vi "PID_model_02.vi"() -> ()   [LabVIEW 2022 SP3]
uses:
  <vilib>/Platform/TimedLoop/XDataNode/timing_clust.ctl
  <vilib>/Platform/TimedLoop/XDataNode/nitl_modes.ctl
  <vilib>/Platform/TimedLoop/XDataNode/wakeup.ctl
  <vilib>/Utility/file.llb/Read Delimited Spreadsheet (DBL).vi
  <vilib>/Platform/TimedLoop/scheduler/LVUserAPI/_suppVIs/Create_1kHz_TSource.vi
  <vilib>/platform/TimedLoop/XDataNode/XDataNode.xnode
  <vilib>/Platform/TimedLoop/XDataNode/XDNodeRunTimeDep.lvlib
  <vilib>/addons/control/pid/NI_PID_pid.lvlib
  <vilib>/gmath/NI_Gmath.lvlib
  <vilib>/addons/control/pid/pid.llb/PID (DBL).vi
panel:
  in  "method":i32(ring)=1 items=["nearest", "linear", "spline", "cubic Hermite", "Lagrange"]
  in  "cluster 2":T1={"Initial X Axis Value"=0, "X Axis Increment"=6.10352, []}
  in  "Setpoint 2":dbl
  in  "Proportional Gain 2":dbl
  in  "method 2":i32(ring)=1 items=["nearest", "linear", "spline", "cubic Hermite", "Lagrange"]
  in  "stop":bool
  out "Plant Output":dbl[](graph)
  in  "cluster":T1={"Initial X Axis Value"=0, "X Axis Increment"=6.10352, []}
  out "Excitation & Response FRFs":T2(graph)
  out "Phase 2":cluster{"Array":dbl[], "Array":dbl[]}(graph) caption="Amplitude [Hz]"
  in  "Skip First N Lines 2":i32=48
  out "Magnitude 2":cluster{"Array":dbl[], "Array":dbl[]}(graph) caption="Amplitude [Hz]"
  out "number of rows 2":i32
  in  "name or relative path 2":path=path "C:/Users/LAV-UFSC/OneDrive - UFSC/Documents/LAV - TCC/Dados-Experimentos/25-04/frf_8.txt"
  out "Phase":cluster{"Array":dbl[], "Array":dbl[]}(graph) caption="Amplitude [Hz]"
  in  "Skip First N Lines":i32=48
  out "Magnitude":cluster{"Array":dbl[], "Array":dbl[]}(graph) caption="Amplitude [Hz]"
  out "number of rows":i32
  in  "name or relative path":path=path "C:/Users/LAV-UFSC/OneDrive - UFSC/Documents/LAV - TCC/Dados-Experimentos/25-04/frf_3.txt"
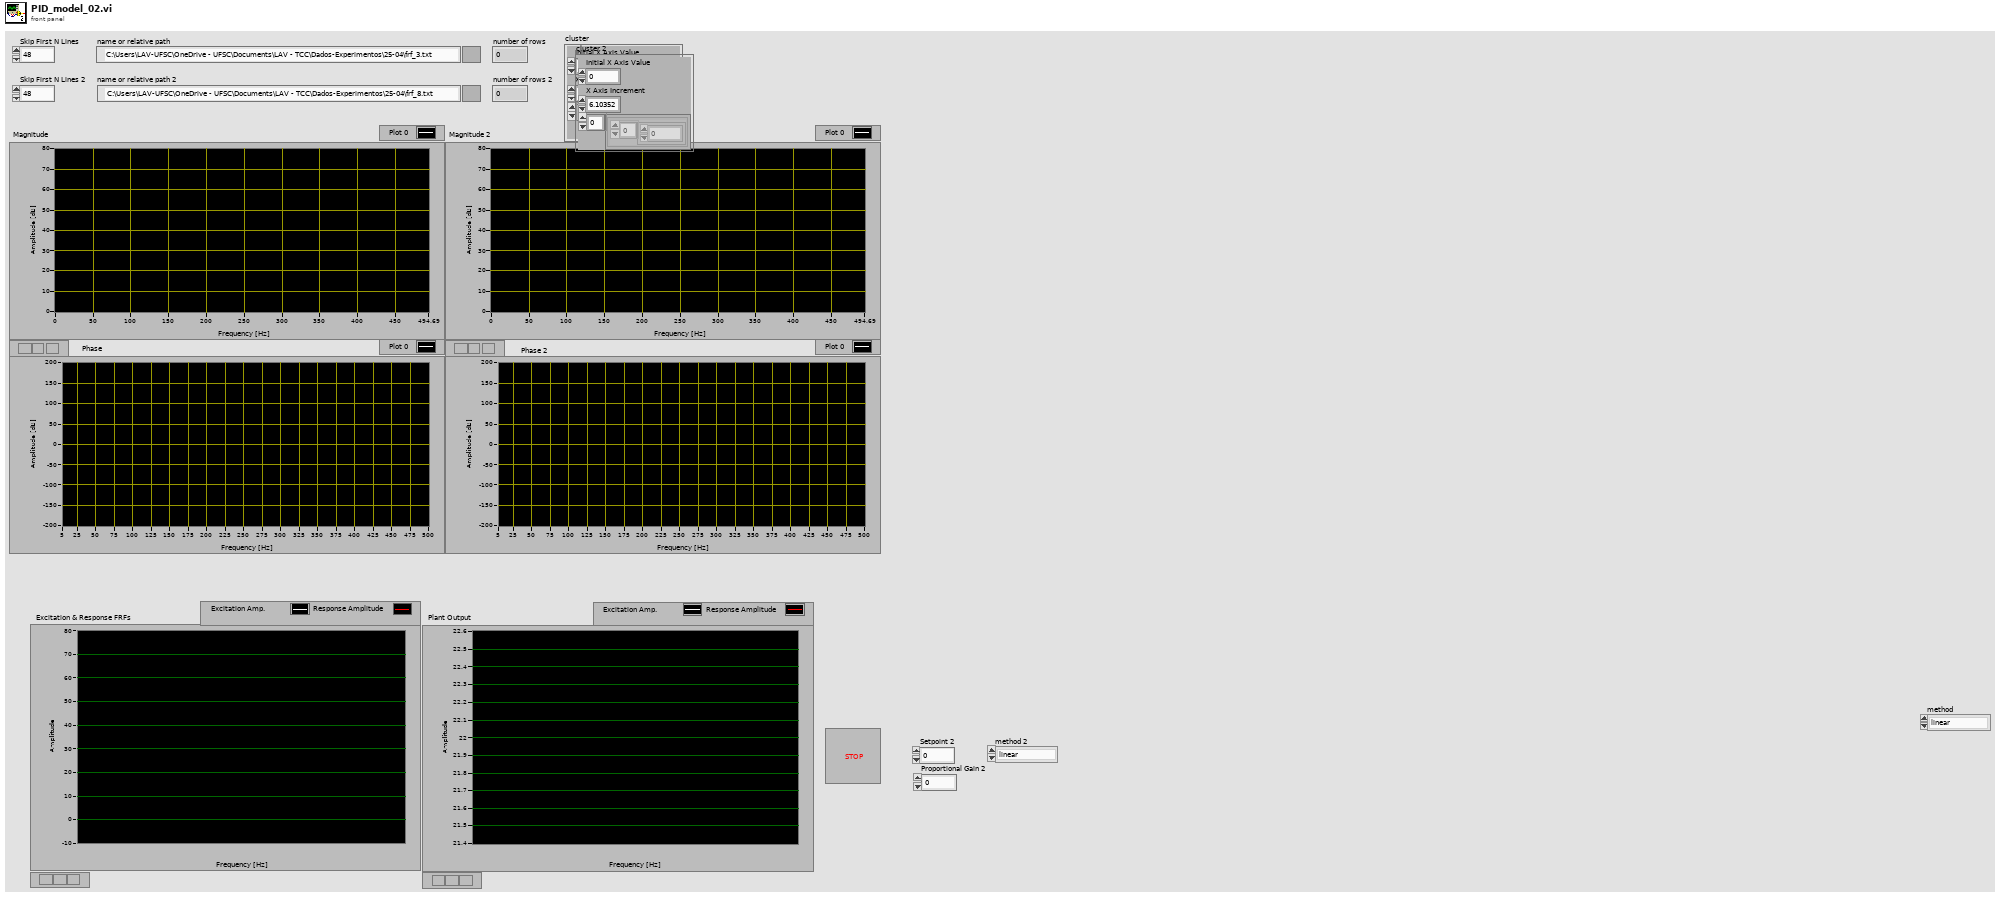
[diagram p1: front panel]
types:
  T1 = cluster{"Initial X Axis Value":i32, "X Axis Increment":dbl, cluster{dbl[]}[]}
  T2 = cluster{i32, "X Axis Increment":dbl, cluster{dbl[]}[]}
  T3 = typedef "XDNodeRunTimeDep.lvlib/timing_clust.ctl" = cluster{"Expected End [f-1]":u64, "Actual End [f-1]":u64, "Finished Late? [f-1]":bool, "Expected End [i-1]":u64, "Actual End [i-1]":u64, "Finished Late? [i-1]":bool, "Expected Start [i]":u64, "Actual Start [i]":u64, "Expected Start [f]":u64, "Actual Start [f]":u64, "Source Name":string, "Structure Name":string, "Period":i64, "Deadline":i64, "Offset":i64, "Start":i64, "Priority":i32, "Timeout":i32, "Mode":T4, "Wakeup Reason":T5, "Error":errorcluster, "Source Type":string, "Secondary Source Type":string, "Global End Time":u64, "Global Start Time":u64, "Frame Duration":u64, "Iteration Duration":u64, "Assigned CPU":i32, "I/O Scan Engine Mode":u32}
  T4 = typedef "XDNodeRunTimeDep.lvlib/nitl_modes.ctl" = enum32{"No Change", "Process missed periods, maintain original phase", "Discard missed periods, maintain original phase", "Process missed periods, ignore original phase", "Discard missed periods, ignore original phase"}
  T5 = typedef "XDNodeRunTimeDep.lvlib/wakeup.ctl" = enum32{"Normal", "Aborted", "Asynchronous wakeup", "Timing source error", "Timed loop error", "Timeout"}
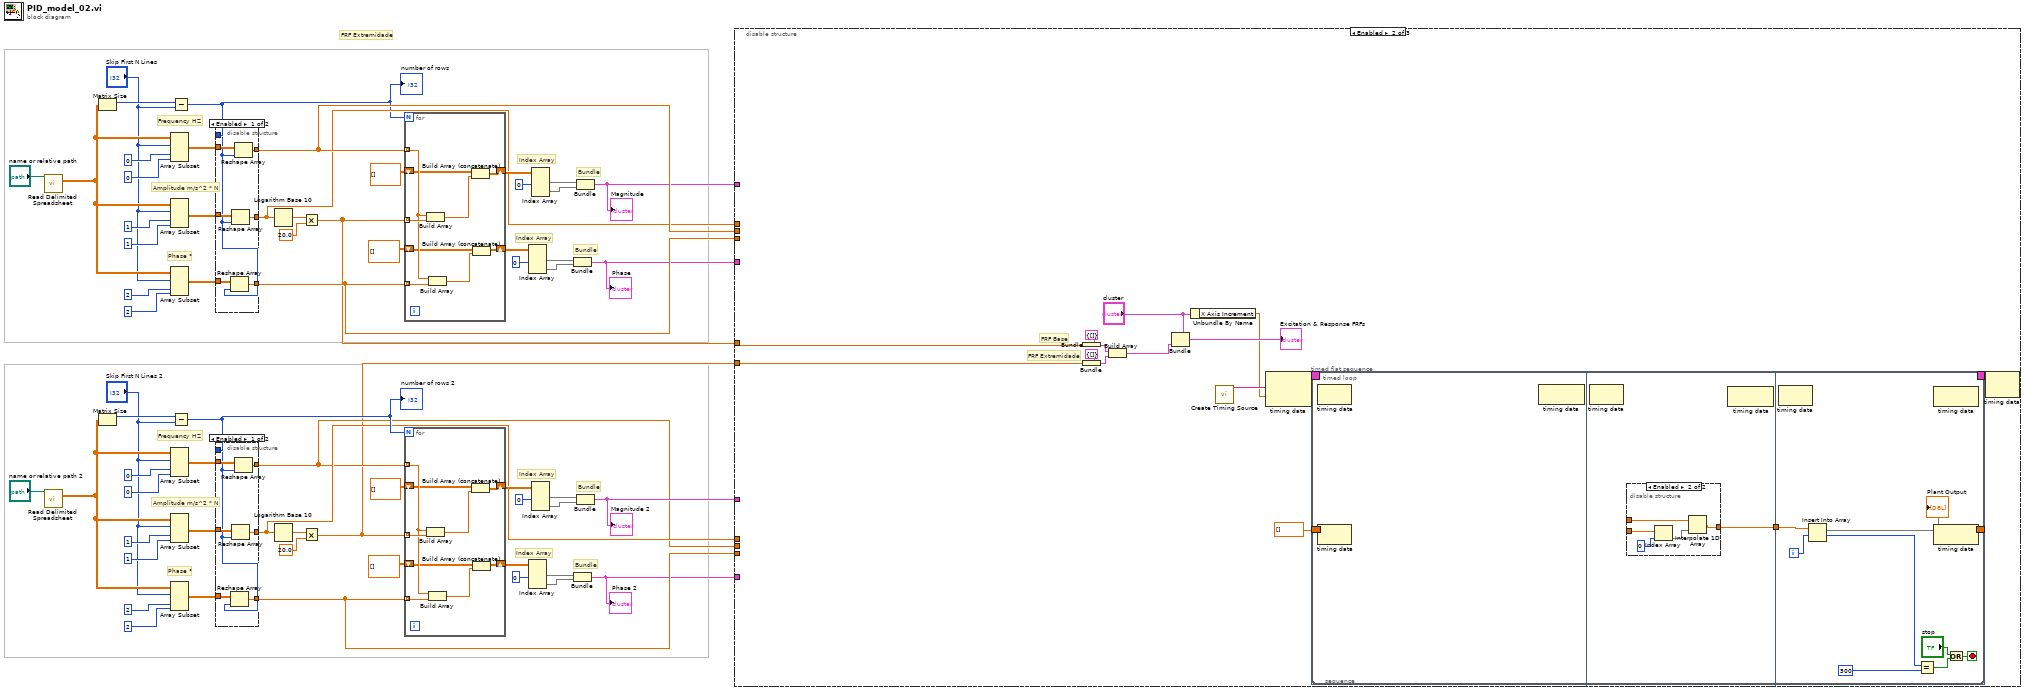
[diagram p0: block diagram]
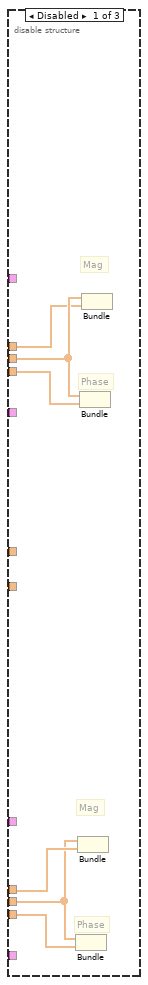
[diagram p3: hidden frame]
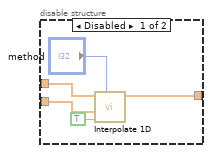
[diagram p4: hidden frame]
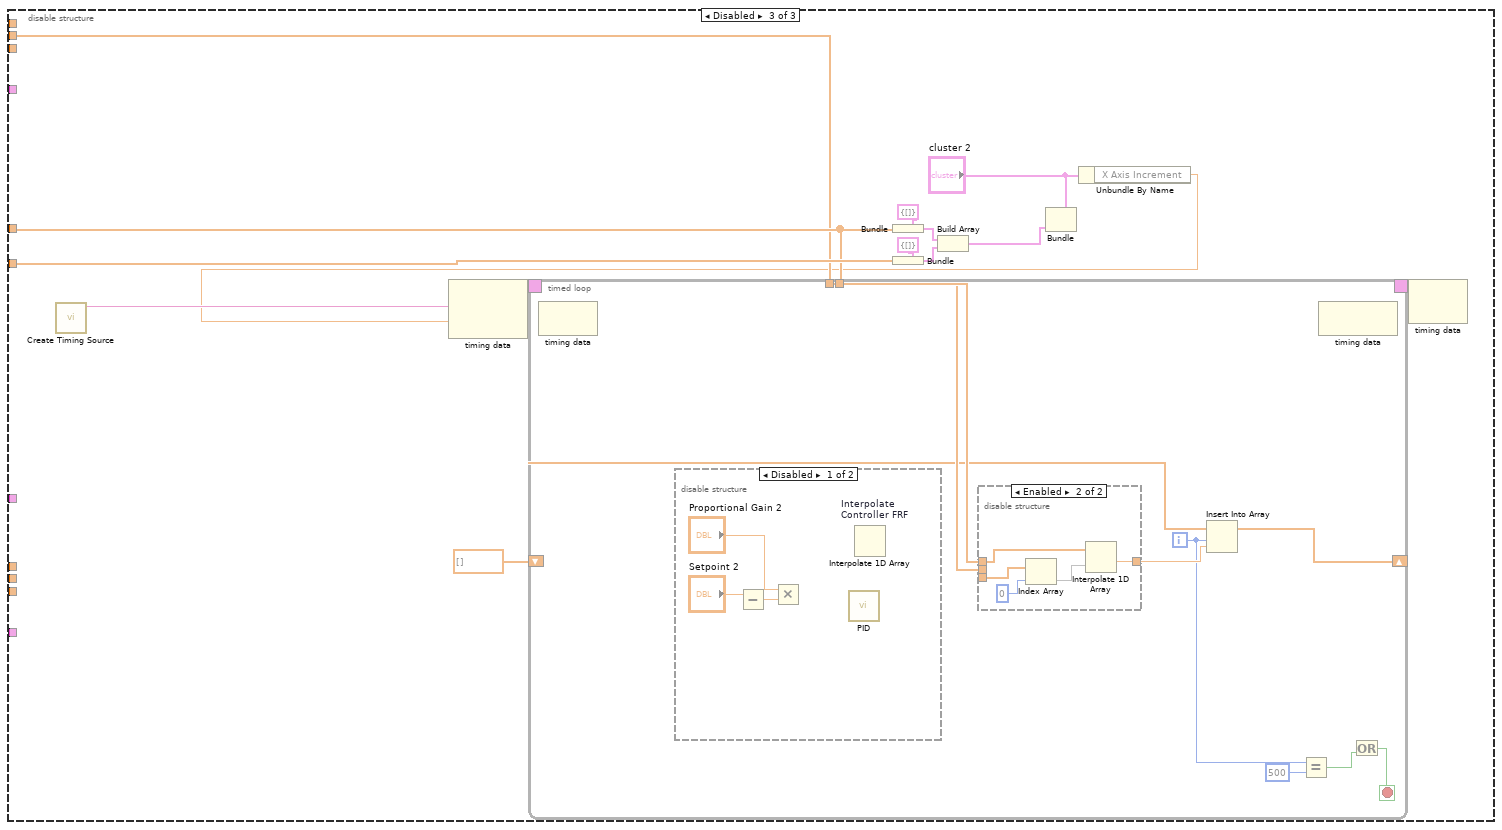
[diagram p5: hidden frame]
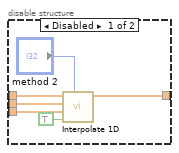
[diagram p6: hidden frame]
diagram:
  # "Index Array"
  # "Bundle"
  # "Index Array"
  # "Bundle"
  # "Phase °"
  # "Amplitude m/s^2 * N"
  # "Frequency HZ"
  # "FRF Extremidade"
  # "Index Array"
  # "Bundle"
  # "Index Array"
  # "Bundle"
  # "Phase °"
  # "Amplitude m/s^2 * N"
  # "Frequency HZ"
  n1 = call-poly <vilib>:"Read Delimited Spreadsheet.vi"("file path (dialog if empty)"="name or relative path") -> ("all rows"=w55:dbl[][])  [unwired: 9 in, 5 out]
  n2 = call-poly <vilib>:"Read Delimited Spreadsheet.vi"("file path (dialog if empty)"="name or relative path 2") -> ("all rows"=w24:dbl[][])  [unwired: 9 in, 5 out]
  n3 = Matrix Size(0:w55) -> (1:w38:i32)  [unwired: 1 out]
  n4 = Matrix Size(0:w24) -> (1:w10:i32)  [unwired: 1 out]
  n5 = Array Subset(array=w55, index (row)="Skip First N Lines", index (col)=0 ("column 1"), length (col)=0 ("column N")) -> (w57:dbl[][])  [unwired: 1 in]
  n6 = Array Subset(array=w55, index (row)="Skip First N Lines", index (col)=1 ("column 1"), length (col)=1 ("column N")) -> (w56:dbl[][])  [unwired: 1 in]
  n7 = Array Subset(array=w55, index (row)="Skip First N Lines", index (col)=2 ("column 1"), length (col)=2 ("column N")) -> (w40:dbl[][])  [unwired: 1 in]
  n8 = Array Subset(array=w24, index (row)="Skip First N Lines 2", index (col)=0 ("column 1"), length (col)=0 ("column N")) -> (w26:dbl[][])  [unwired: 1 in]
  n9 = Array Subset(array=w24, index (row)="Skip First N Lines 2", index (col)=1 ("column 1"), length (col)=1 ("column N")) -> (w25:dbl[][])  [unwired: 1 in]
  n10 = Array Subset(array=w24, index (row)="Skip First N Lines 2", index (col)=2 ("column 1"), length (col)=2 ("column N")) -> (w11:dbl[][])  [unwired: 1 in]
  n11 = Subtract(x=w38, y="Skip First N Lines") -> (x-y=w36:i32)
  "number of rows" <- w36
  n12 = Subtract(x=w10, y="Skip First N Lines 2") -> (x-y=w8:i32)
  "number of rows 2" <- w8
  n13 = disable-structure shown="Enabled" {
    disable-tunnel: w57 -> [w71 w73]
    disable-tunnel: w56 -> [w70 w72]
    disable-tunnel: [w69 w73] -> w42
    disable-tunnel: [w68 w72] -> w41
    disable-tunnel: w36 -> [w66 _]
    disable-tunnel: w40 -> [w67 _]
    disable-tunnel: [w65 _] -> w39
    frame Enabled {
      n14 = Reshape Array(w67, w66) -> (w65:dbl[])
      n15 = Reshape Array(w70, w66) -> (w68:dbl[])
      n16 = Reshape Array(w71, w66) -> (w69:dbl[])
    }
    frame Disabled {
    }
  }
  n17 = disable-structure shown="Enabled" {
    disable-tunnel: w26 -> [w80 w82]
    disable-tunnel: w25 -> [w79 w81]
    disable-tunnel: [w78 w82] -> w5
    disable-tunnel: [w77 w81] -> w6
    disable-tunnel: w8 -> [w75 _]
    disable-tunnel: w11 -> [w76 _]
    disable-tunnel: [w74 _] -> w4
    frame Enabled {
      n18 = Reshape Array(w76, w75) -> (w74:dbl[])
      n19 = Reshape Array(w79, w75) -> (w77:dbl[])
      n20 = Reshape Array(w80, w75) -> (w78:dbl[])
    }
    frame Disabled {
    }
  }
  n21 = Logarithm Base 10(1:w41) -> (0:w48:dbl[])
  n22 = Logarithm Base 10(1:w6) -> (0:w17:dbl[])
  n23 = Multiply(x=w48, y=20.0) -> (x*y=w1:dbl[])
  n24 = Multiply(x=w17, y=20.0) -> (x*y=w2:dbl[])
  n25 = for {
    N: w36 -> [_]
    tunnel: w42 -> [w89] mode=indexing
    tunnel: w1 -> [w90] mode=indexing
    tunnel: w39 -> [w91] mode=indexing
    shift-right: [w86] -> w50
    shift-left: dbl[][] [] -> [w88]
    shift-right: [w85] -> w43
    shift-left: dbl[][] [] -> [w84]
    n26 = Build Array(w89, w90) -> (w87:dbl[])
    n27 = Build Array(w89, w91) -> (w83:dbl[])
    n28 = Build Array (concatenate)(w88, w87) -> (w86:dbl[][])
    n29 = Build Array (concatenate)(w84, w83) -> (w85:dbl[][])
  }
  n30 = for {
    N: w8 -> [_]
    tunnel: w5 -> [w98] mode=indexing
    tunnel: w2 -> [w99] mode=indexing
    tunnel: w4 -> [w100] mode=indexing
    shift-right: [w95] -> w19
    shift-left: dbl[][] [] -> [w97]
    shift-right: [w94] -> w12
    shift-left: dbl[][] [] -> [w93]
    n31 = Build Array(w98, w99) -> (w96:dbl[])
    n32 = Build Array(w98, w100) -> (w92:dbl[])
    n33 = Build Array (concatenate)(w97, w96) -> (w95:dbl[][])
    n34 = Build Array (concatenate)(w93, w92) -> (w94:dbl[][])
  }
  n35 = Index Array(array=w43, index (col) #1=0 ("disabled index (col)")) -> (element #1=w44:dbl[], element #2=w45:dbl[])  [unwired: 3 in]
  n36 = Index Array(array=w12, index (col) #1=0 ("disabled index (col)")) -> (element #1=w13:dbl[], element #2=w14:dbl[])  [unwired: 3 in]
  n37 = Index Array(array=w50, index (col) #1=0 ("disabled index (col)")) -> (element #1=w51:dbl[], element #2=w52:dbl[])  [unwired: 3 in]
  n38 = Index Array(array=w19, index (col) #1=0 ("disabled index (col)")) -> (element #1=w20:dbl[], element #2=w21:dbl[])  [unwired: 3 in]
  n39 = Bundle(w44, w45) -> (w34:cluster{dbl[], dbl[]})  [unwired: 1 in]
  "Phase" <- w34
  n40 = Bundle(w13, w14) -> (w3:cluster{dbl[], dbl[]})  [unwired: 1 in]
  "Phase 2" <- w3
  n41 = Bundle(w51, w52) -> (w35:cluster{dbl[], dbl[]})  [unwired: 1 in]
  "Magnitude" <- w35
  n42 = Bundle(w20, w21) -> (w7:cluster{dbl[], dbl[]})  [unwired: 1 in]
  "Magnitude 2" <- w7
  n43 = disable-structure shown="Enabled" {
    disable-tunnel: w42 -> [w106 _ w162]
    disable-tunnel: w41 -> [w105 _ _]
    disable-tunnel: w39 -> [w104 _ _]
    disable-tunnel: w35 -> [_ _ _]
    disable-tunnel: w34 -> [_ _ _]
    disable-tunnel: w7 -> [_ _ _]
    disable-tunnel: w6 -> [w103 _ _]
    disable-tunnel: w5 -> [w101 _ _]
    disable-tunnel: w4 -> [w102 _ _]
    disable-tunnel: w3 -> [_ _ _]
    disable-tunnel: w2 -> [_ w116 w168]
    disable-tunnel: w1 -> [_ w113 w165]
    frame Disabled {
      # "Phase"
      # "Mag"
      # "Phase"
      # "Mag"
      n44 = Bundle("all rows"=w101, "all rows"=w102) -> ()  [unwired: 2 out]
      n45 = Bundle("all rows"=w101, "all rows"=w103) -> ()  [unwired: 2 out]
      n46 = Bundle("all rows"=w106, "all rows"=w104) -> ()  [unwired: 2 out]
      n47 = Bundle("all rows"=w106, "all rows"=w105) -> ()  [unwired: 2 out]
    }
    frame Enabled {
      # "FRF Base"
      # "FRF Extremidade"
      n48 = Bundle(cluster=cluster{dbl[]} {[]} ("Excitation Amplitude [dB]"), w113) -> (w120:cluster{dbl[]})
      n49 = Bundle(cluster=cluster{dbl[]} {[]} ("Response Amplitude [dB]"), w116) -> (w119:cluster{dbl[]})
      n50 = Build Array(w120, w119) -> (w118:cluster{dbl[]}[])
      n51 = Bundle(cluster="cluster", w118) -> (→"Excitation & Response FRFs":T1)  [unwired: 2 in]
      n52 = Unbundle By Name("cluster") -> ("X Axis Increment"=w108:dbl)
      n53 = call-poly <vilib>:"Create Timing Source.vi"() -> ("name (out)"=w109:string)  [unwired: 10 in, 1 out]
      n54 = node-c288(w109, w108) -> (w112:T3)
      n55 = timed-loop {
        timing: w112 -> [_]
        timing-out: [_] -> w111
        shift-right: [w121] -> _
        shift-left: dbl[] [] ("yi") -> [w122]
        i -> [w147]
        stop <- w144 stop-if-true
        n56 = timed-sequence {
          timing: _ -> [_]
          timing-out: _ -> [_]
          tunnel: w122 -> [w125]
          tunnel: [w124] -> w121
          n57 = timed-flat-sequence {
            tunnel: w125 -> [_]
            tunnel: [w128] -> w123
            tunnel: [w143] -> w124
            tunnel: w123 -> [w142]
            frame #0 {
              n58 = node-c288() -> ()  [unwired: 1 in, 1 out]
              n59 = node-c288() -> ()  [unwired: 1 in, 1 out]
            }
            frame #1 {
              n60 = node-c288() -> ()  [unwired: 1 in, 1 out]
              n61 = disable-structure shown="Enabled" {
                disable-tunnel: _ -> [w134 w138]
                disable-tunnel: _ -> [w131 w137]
                disable-tunnel: [w130 w139] -> w128
                frame Disabled {
                  n62 = call <vilib>:"Interpolate 1D.vi"("method"="method", "X is monotonic"=TRUE, "xi"=w131, "Y"=w134) -> ("yi"=w130:dbl[], "X"=w133:dbl[])  [unwired: 4 in, 2 out]
                }
                frame Enabled {
                  n63 = Index Array(array=w137, index=0) -> (element=w135)
                  n64 = Interpolate 1D Array(1:w135, 2:w138) -> (0:w139:dbl)
                }
              }
              n65 = node-c288() -> ()  [unwired: 1 in, 1 out]
            }
            frame #2 {
              n66 = node-c288() -> ()  [unwired: 1 in, 1 out]
              n67 = Insert Into Array(array=w142, index=w147) -> (w143)  [unwired: 1 in]
              "Plant Output" <- w143
              n68 = Equal?(x=w147, y=500) -> (x = y?=w146:bool)
              n69 = node-c288() -> ()  [unwired: 1 in, 1 out]
              n70 = Or(x="stop", y=w146) -> (x .or. y?=w144:bool)
            }
          }
        }
        n71 = node-c288() -> ()  [unwired: 1 in, 1 out]
        n72 = node-c288() -> ()  [unwired: 1 in, 1 out]
      }
      n73 = node-c288(w111) -> ()  [unwired: 1 out]
    }
    frame Disabled {
      n74 = call-poly <vilib>:"Create Timing Source.vi"() -> ("name (out)"=w160:string)  [unwired: 10 in, 1 out]
      n75 = Bundle(cluster=cluster{dbl[]} {[]} ("Excitation Amplitude [dB]"), w165) -> (w172:cluster{dbl[]})
      n76 = Bundle(cluster=cluster{dbl[]} {[]} ("Response Amplitude [dB]"), w168) -> (w171:cluster{dbl[]})
      n77 = Build Array(w172, w171) -> (w170:cluster{dbl[]}[])
      n78 = Bundle(cluster="cluster 2", w170) -> (w169:T1)  [unwired: 2 in]
      n79 = Unbundle By Name("cluster 2") -> ("X Axis Increment"=w159:dbl)
      n80 = node-c288(w160, w159) -> (w164:T3)
      n81 = timed-loop {
        tunnel: w165 -> [w181]
        timing: w164 -> [_]
        timing-out: [_] -> w163
        tunnel: w162 -> [w180]
        shift-right: [w178] -> _
        shift-left: dbl[] [] ("yi") -> [w179]
        i -> [w174]
        stop <- w176 stop-if-true
        n82 = node-c288() -> ()  [unwired: 1 in, 1 out]
        n83 = disable-structure shown="Disabled" {
          frame Disabled {
            n84 = Subtract(x="Setpoint 2") -> (y=w193:dbl, x-y=w195:dbl)
            n85 = Multiply(x="Proportional Gain 2", y=w195) -> ()  [unwired: 1 out]
            n86 = call-poly <vilib>:"PID.vi"() -> ()  [unwired: 10 in, 2 out]
            n87 = Interpolate 1D Array "Interpolate\nController FRF"() -> ()  [unwired: 2 in, 1 out]
          }
          frame Enabled {
          }
        }
        n88 = disable-structure shown="Enabled" {
          disable-tunnel: w181 -> [w187 w191]
          disable-tunnel: w180 -> [w186 _]
          disable-tunnel: _ -> [w184 w190]
          disable-tunnel: [w183 w192] -> w177
          frame Disabled {
            n89 = call <vilib>:"Interpolate 1D.vi"("method"="method 2", "X is monotonic"=TRUE, "xi"=w184, "X"=w186, "Y"=w187) -> ("yi"=w183:dbl[])  [unwired: 4 in, 2 out]
          }
          frame Enabled {
            n90 = Index Array(array=w190, index=0) -> (element=w188)
            n91 = Interpolate 1D Array(1:w188, 2:w191) -> (0:w192:dbl)
          }
        }
        n92 = Insert Into Array(array=w179, index=w174, new element=w177) -> (w178:dbl[])
        n93 = Equal?(x=w174, y=500) -> (x = y?=w175:bool)
        n94 = node-c288() -> ()  [unwired: 1 in, 1 out]
        n95 = Or(y=w175) -> (x .or. y?=w176:bool)  [unwired: 1 in]
      }
      n96 = node-c288(w163) -> ()  [unwired: 1 out]
    }
  }
